vi "MQTT_Connect.vi"(5 "Connect Meta":T5={"QoS"=enum."At most once", "DUP"=FALSE, "Retain"=TRUE, "Keep Alive (sec)"=60}, 6 "Client ID":string="NodeE-12345", 7 "Connect Flags":T8={"user name"=FALSE, "password"=FALSE, "will retain"=TRUE, "will flag"=FALSE, "clean session"=FALSE, "reserved"=FALSE, "will QoS"=enum."At most once"}, 8 "error in (no error)":errorcluster, 9 "Will Info":T6={"Will message"="Last Will", "Will Topic"="Will Topic"}, 10 "User Info":T7={"User Name"="User", "Password"="password"}, 11 "MQTT Broker":cluster{"address (IP)":string, "port":u16}={"address (IP)"="broker.mqttdashboard.com", "port"=1883}) -> (0 "error out":errorcluster, 2 "Connection Status":T1=enum."Connection refused: not authorized", 3 "connection ID out":refnum<k5>)   [LabVIEW 2015, in "MQTT_Functions.lvlib"]
uses:
  MQTT_Functions.lvlib
  Controls/Connect_Flags.ctl
  Controls/QoS.ctl
  Controls/User_Info.ctl
  Controls/Will_Info.ctl
  Controls/DUP_Flag.ctl
  Controls/Retain_Flag.ctl
  Controls/Connection_Return_Codes.ctl
  Controls/MessageType.ctl
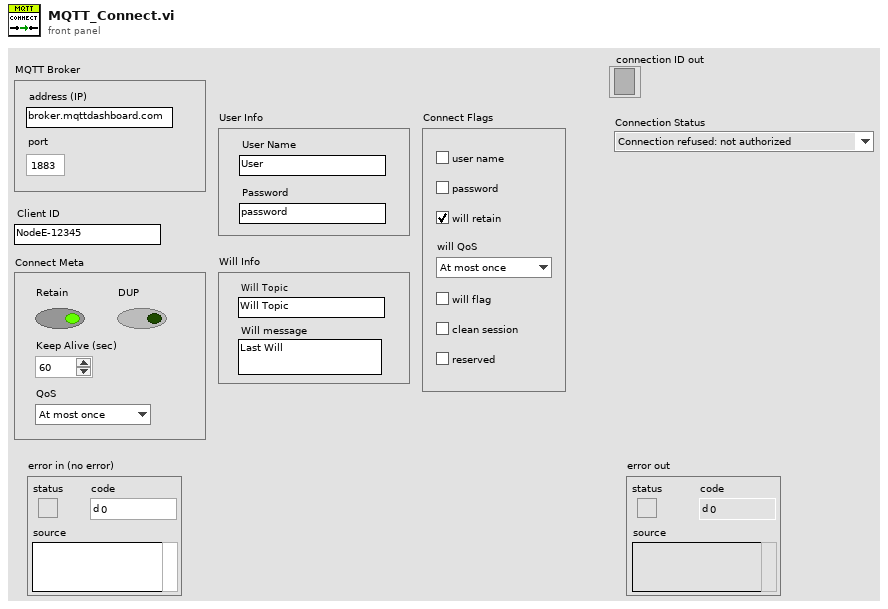
[diagram p1: front panel]
types:
  T1 = typedef "MQTT_Functions.lvlib/Connection_Return_Codes.ctl" = enum16{"Connection accepted", "Connection refused: unacceptable protocol version", "Connection refused: identifier rejected", "Connection refused: Server unavailable", "Connection refused: bad user name or password", "Connection refused: not authorized"}
  T2 = typedef "MQTT_Functions.lvlib/QoS.ctl" = enum8{"At most once", "At least once", "Exactly once", "Reserved"}
  T3 = typedef "MQTT_Functions.lvlib/DUP_Flag.ctl" = bool
  T4 = typedef "MQTT_Functions.lvlib/Retain_Flag.ctl" = bool
  T5 = cluster{"QoS":T2, "DUP":T3, "Retain":T4, "Keep Alive (sec)":u16}
  T6 = typedef "MQTT_Functions.lvlib/Will_Info.ctl" = cluster{"Will message":string, "Will Topic":string}
  T7 = typedef "MQTT_Functions.lvlib/User_Info.ctl" = cluster{"User Name":string, "Password":string}
  T8 = typedef "MQTT_Functions.lvlib/Connect_Flags.ctl" = cluster{"user name":bool, "password":bool, "will retain":bool, "will flag":bool, "clean session":bool, "reserved":bool, "will QoS":T2}
  T9 = typedef "MQTT_Functions.lvlib/MessageType.ctl" = enum32{"Reserved", "CONNECT", "CONNACK", "PUBLISH", "PUBACK", "PUBREC", "PUBREL", "PUBCOMP", "SUBSCRIBE", "SUBACK", "UNSUBSCRIBE", "UNSUBACK", "PINGREQ", "PINGRESP", "DISCONNECT", "Reserved2"}
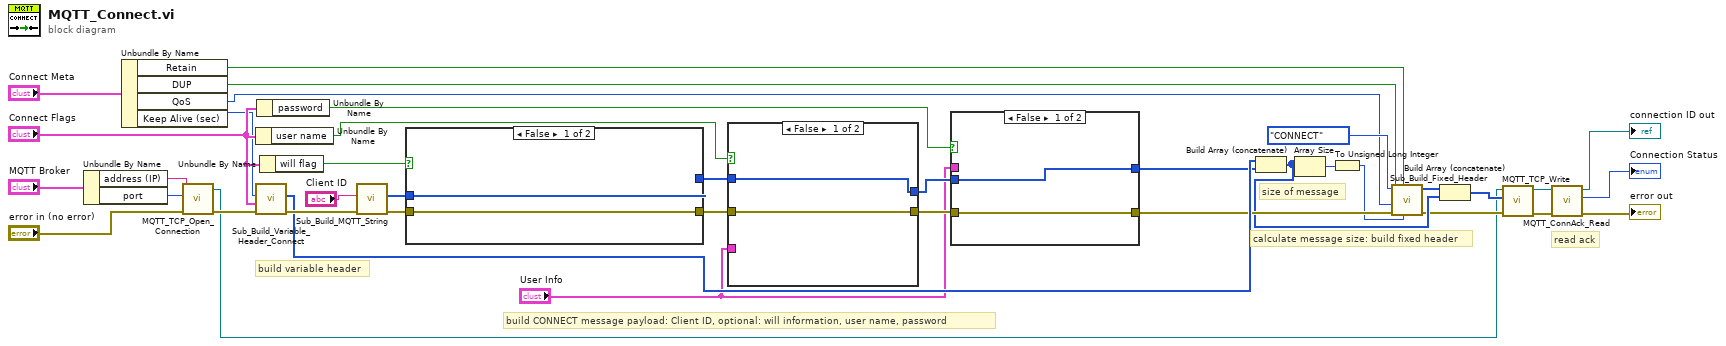
[diagram p0: block diagram]
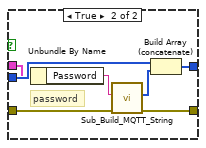
[diagram p2: hidden frame]
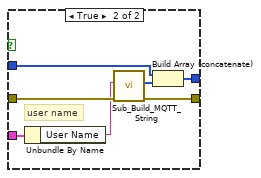
[diagram p3: hidden frame]
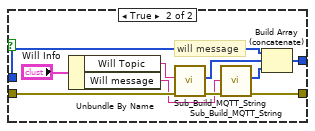
[diagram p4: hidden frame]
diagram:
  # "read ack"
  # "calculate message size: build fixed header"
  # "build CONNECT message payload: Client ID, optional: will information, user name, password"
  # "build variable header"
  # "size of message"
  n1 = Unbundle By Name("MQTT Broker") -> ("address (IP)"=w7:string, "port"=w1:u16)
  n2 = Unbundle By Name("Connect Meta") -> ("Retain"=w18:T4, "DUP"=w17:T3, "QoS"=w16:T2, "Keep Alive (sec)"=w15:u16)
  n3 = call "MQTT_TCP_Open_Connection.vi"("error in (no error)"="error in (no error)", "remote port or service name"=w1, "address"=w7) -> ("error out"=w10:errorcluster, "connection ID"=w9:refnum<k5>)  [unwired: 7 in]
  n4 = Unbundle By Name("Connect Flags") -> ("user name"=w32:bool)
  n5 = call "Sub_Build_Variable_Header_Connect.vi"("error in (no error)"=w10, "Connect Flags"="Connect Flags", "Keep Alive (sec)"=w15) -> ("error out"=w38:errorcluster, "Variable Header"=w29:u8[])  [unwired: 7 in]
  n6 = Unbundle By Name("Connect Flags") -> ("password"=w31:bool)
  n7 = Unbundle By Name("Connect Flags") -> ("will flag"=w30:bool)
  n8 = call "Sub_Build_MQTT_String.vi"("error in (no error)"=w38, "String to be encoded"="Client ID") -> ("error out"=w34:errorcluster, "UTF8 Byte Array"=w37:u8[])  [unwired: 8 in]
  n9 = case shown="False" w30 {
    tunnel: w37 -> [w41 w49]
    tunnel: [w41 w50] -> w36
    tunnel: w34 -> [w40 w48]
    tunnel: [w40 w45] -> w27
    frame False {
    }
    frame True {
      # "will message"
      n10 = Unbundle By Name("Will Info") -> ("Will Topic"=w43:string, "Will message"=w42:string)
      n11 = call "Sub_Build_MQTT_String.vi"("error in (no error)"=w48, "String to be encoded"=w43) -> ("error out"=w47:errorcluster, "UTF8 Byte Array"=w46:u8[])  [unwired: 8 in]
      n12 = call "Sub_Build_MQTT_String.vi"("error in (no error)"=w47, "String to be encoded"=w42) -> ("error out"=w45:errorcluster, "UTF8 Byte Array"=w51:u8[])  [unwired: 8 in]
      n13 = Build Array (concatenate)(w49, w46, w51) -> (w50:u8[])
    }
  }
  n14 = case shown="False" w32 {
    tunnel: w36 -> [w53 w59]
    tunnel: [w53 w58] -> w35
    tunnel: [w52 w57] -> w28
    tunnel: w27 -> [w52 w56]
    tunnel: "User Info" -> [_ w55]
    frame False {
    }
    frame True {
      # "user name"
      n15 = Unbundle By Name(w55) -> ("User Name"=w54:string)
      n16 = call "Sub_Build_MQTT_String.vi"("error in (no error)"=w56, "String to be encoded"=w54) -> ("error out"=w57:errorcluster, "UTF8 Byte Array"=w60:u8[])  [unwired: 8 in]
      n17 = Build Array (concatenate)(w59, w60) -> (w58:u8[])
    }
  }
  n18 = case shown="False" w31 {
    tunnel: w35 -> [w62 w68]
    tunnel: [w62 w67] -> w25
    tunnel: w28 -> [w61 w66]
    tunnel: [w61 w65] -> w26
    tunnel: "User Info" -> [_ w64]
    frame False {
    }
    frame True {
      # "password"
      n19 = Unbundle By Name(w64) -> ("Password"=w63:string)
      n20 = call "Sub_Build_MQTT_String.vi"("error in (no error)"=w66, "String to be encoded"=w63) -> ("error out"=w65:errorcluster, "UTF8 Byte Array"=w69:u8[])  [unwired: 8 in]
      n21 = Build Array (concatenate)(w68, w69) -> (w67:u8[])
    }
  }
  n22 = Build Array (concatenate)(w29, w25) -> (w24:u8[])
  n23 = Array Size(array=w24) -> (size(s)=w22:i32)
  n24 = To Unsigned Long Integer(number=w22) -> (unsigned 32bit integer=w21:u32)
  n25 = call "Sub_Build_Fixed_Header.vi"("Remaining Length"=w21, "Retain"=w18, "error in (no error)"=w26, "QoS"=w16, "DUP"=w17, "MessageType"=MessageType."CONNECT") -> ("error out"=w13:errorcluster, "Fixed Header"=w23:u8[])  [unwired: 4 in]
  n26 = Build Array (concatenate)(w23, w24) -> (w12:u8[])
  n27 = call "MQTT_TCP_Write.vi"("error in (no error)"=w13, "data in"=w12, "connection ID"=w9) -> ("error out"=w6:errorcluster, "connection ID out"=w5:refnum<k5>)  [unwired: 6 in, 1 out]
  n28 = call "MQTT_ConnAck_Read.vi"("error in (no error)"=w6, "connection ID"=w5) -> ("error out"=→"error out":errorcluster, "Connection Status"=→"Connection Status":T1, "connection ID out"=→"connection ID out":refnum<k5>)  [unwired: 5 in, 2 out]
